vi "Init Node Info.vi"(8 "error in (no error)":errorcluster, 11 "DiscoveryService in":refnum<class "NodeDiscovery.lvclass">) -> (0 "error out":errorcluster, 3 "DiscoveryService out":refnum<class "NodeDiscovery.lvclass">)   [LabVIEW 2020, in "Vecto.lvlib" / "NodeDiscovery.lvclass"]
uses:
  NodeDiscovery.lvclass
  proto/ServiceType/Enumeration.ctl
  proto/ServiceType/ServiceType.lvlib
  proto/Service/Data.ctl
  proto/Service/Service.lvlib
  proto/Discovery/Data.ctl
  proto/Discovery/Discovery.lvlib
  Node Config/Node Config.lvclass
  proto/Discovery/Class/Msg.lvclass
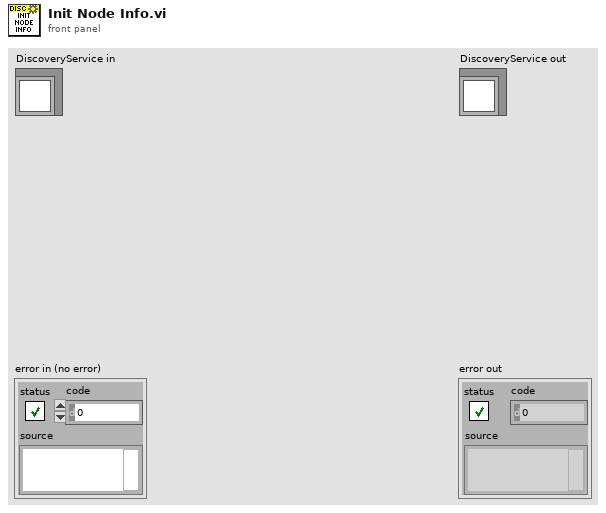
[diagram p1: front panel]
types:
  T1 = typedef "Discovery.lvlib/Data.ctl" = cluster{"node_id":u32, "name":string, "ip":u32, "status":string, "services":T2[], "system":string, "cluster":string}
  T2 = typedef "Service.lvlib/Data.ctl" = cluster{"type":T3, "port":i32}
  T3 = typedef "ServiceType.lvlib/Enumeration.ctl" = enum16{"SERVICETYPE_UNKNOWN", "SERVICETYPE_TCPSERVER", "SERVICETYPE_HTTPSERVER"}
  T4 = typedef "Vecto.lvlib/Node Config.lvclass/Discovery Info.ctl" = cluster{"Address":string, "Port":u16, "Interval S":dbl, "Bind Address":string}
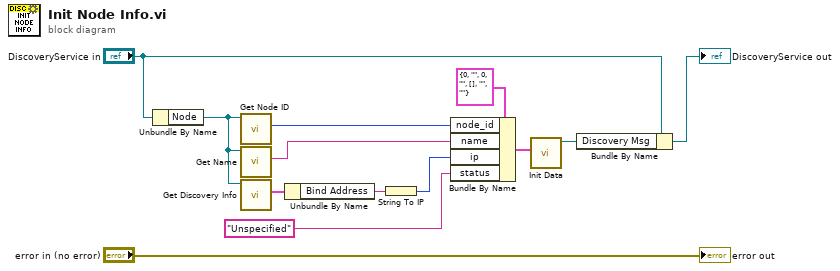
[diagram p0: block diagram]
diagram:
  n1 = Unbundle By Name("DiscoveryService in") -> ("Node"=w5:refnum<class "Node Config.lvclass">)
  n2 = call "Get Node ID.vi"("Node in"=w5) -> ("Node ID"=w12:u32)  [unwired: 8 in, 2 out]
  n3 = call "Get Name.vi"("Node in"=w5) -> ("Name"=w11:string)  [unwired: 8 in, 2 out]
  n4 = call "Get Discovery Info.vi"("Node in"=w5) -> ("Discovery Info"=w2:T4)  [unwired: 8 in, 2 out]
  n5 = Unbundle By Name(w2) -> ("Bind Address"=w1:string)
  n6 = String To IP(1:w1) -> (0:w4:u32)
  n7 = Bundle By Name(cluster=T1 {"node_id"=0, "name"="", "ip"=0, "status"="", "services"=[], "system"="", "cluster"=""} ("Discovery"), "node_id"=w12, "name"=w11, "ip"=w4, "status"="Unspecified") -> (w9:T1)
  n8 = call "Init Data.vi"("Data"=w9) -> ("Msg out"=w7:refnum<class "Msg.lvclass">)  [unwired: 10 in]
  n9 = Bundle By Name(cluster="DiscoveryService in", "Discovery Msg"=w7) -> (→"DiscoveryService out":refnum<class "NodeDiscovery.lvclass">)
  "error out" <- "error in (no error)"
